vi "SetAttributeViInt32_SA-Marker_Source.vi"(7 "AttributeValue":i32 format="%.0g", 8 "error in (no error)":errorcluster {"code" format="%.0x"}, 9 "AttributeID":u32(ring)=1150711 items=["SA_MARKER_ACTIVE_MARKER"=1150711, "SA_MARKER_DELTA_REFERENCE"=1150690, "SA_MARKER_FUNCTION"=1150692, "SA_MARKER_PEAK_SEARCH_MODE"=1150709, "SA_MARKER_PEAK_SORT_MODE"=1150708, "SA_MARKER_PEAK_TABLE_READOUT_MODE"=1150707, "SA_MARKER_TRACE"=1150720, "SA_MARKER_TYPE"=1150721, "SA_MARKER_X_AXIS_SCALE"=1150698, "SA_SOURCE_FREQUENCY_MULTIPLIER_DENOMINATOR"=1150795, "SA_SOURCE_FREQUENCY_MULTIPLIER_NUMERATOR"=1150794, "SA_SOURCE_MODE"=1150799, "SA_SOURCE_POINT_TRIGGER_TYPE"=1150801], 11 "instrument handle":refnum<k15>) -> (0 "error out":errorcluster {"code" format="%.0x"}, 3 "instrument handle out":refnum<k15>)   [LabVIEW 2009, in "Keysight XSAn.lvlib"]
doc: "Sets an Int32 attribute from the instrument driver.\nThe following Attributes are supported:\n\nSA_MARKER_ACTIVE_MARKER\nSA_MARKER_DELTA_REFERENCE\nSA_MARKER_FUNCTION\nSA_MARKER_PEAK_SEARCH_MODE\nSA_MARKER_PEAK_SORT_MODE\nSA_MARKER_PEAK_TABLE_READOUT_MODE\nSA_MARKER_TRACE\nSA_MARKER_TYPE\nSA_MARKER_X_AXIS_SCALE\nSA_SOURCE_FREQUENCY_MULTIPLIER_DENOMINATOR\nSA_SOURCE_FREQUENCY_MULTIPLIER_NUMERATOR\nSA_SOURCE_MODE\nSA_SOURCE_POINT_TRIGGER_TYPE"
uses:
  <instrlib>/Keysight XSAn/Keysight XSAn.lvlib
  AgXSAn.dll
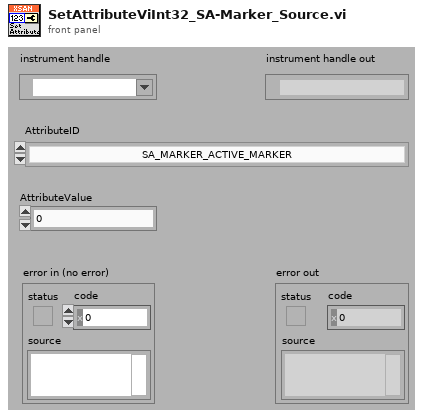
[diagram p1: front panel]
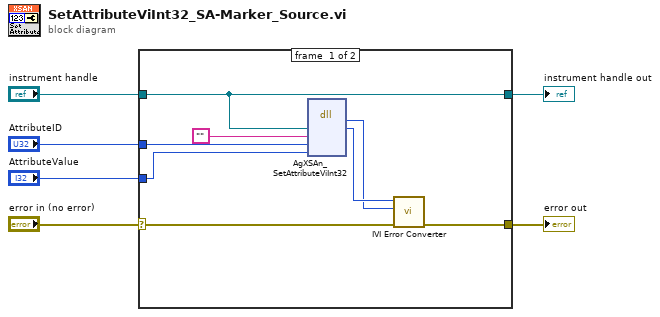
[diagram p0: block diagram]
diagram:
  n1 = case shown="No Error" "error in (no error)" {
    selector: "error in (no error)" -> [w12 w16]
    tunnel: [w11 w16] -> w6
    tunnel: "instrument handle" -> [w8 w15]
    tunnel: "AttributeID" -> [w10 _]
    tunnel: "AttributeValue" -> [w9 _]
    tunnel: [w8 w15] -> w1
    frame #0 {
      n2 = dll-call lib="AgXSAn**.dll" fn="AgXSAn_SetAttributeViInt32"("Vi"=w8, "RepCapIdentifier"="", "AttributeID"=w10, "AttributeValue"=w9) -> ("return type"=w13:i32, "Vi"=w14:u32)  [unwired: 6 in, 2 out]
      n3 = call <instrlib>:"IVI Error Converter.vi"("error in (no error)"=w12, "IVI error code (0)"=w13, "instrument handle"=w14) -> ("error out"=w11:errorcluster)  [unwired: 7 in, 1 out]
    }
    frame #1 {
    }
  }
  "error out" <- w6
  "instrument handle out" <- w1
